vi "forward difference (i32).vi"(3 "Y":i32[](array[numeric])) -> (1 "Y(i+1)-Y(i)":i32[](array[numeric]))   [LabVIEW 2009, in "common.lvlib"]
uses:
  common.lvlib
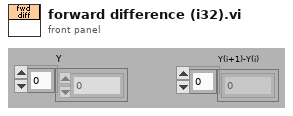
[diagram p1: front panel]
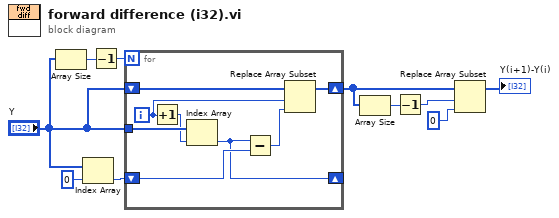
[diagram p0: block diagram]
diagram:
  n1 = Array Size(array="Y") -> (size(s)=w10:i32)
  n2 = Index Array(array="Y", index=0) -> (element=w7:i32)
  n3 = Decrement(x=w10) -> (x-1=w9:i32)
  n4 = for {
    N: w9 -> [_]
    tunnel: "Y" -> [w18]
    shift-right: [w15] -> _
    shift-left: w7 -> [w16]
    shift-right: [w11] -> w4
    shift-left: "Y" -> [w12]
    i -> [w13]
    n5 = Increment(x=w13) -> (x+1=w17:i32)
    n6 = Index Array(array=w18, index=w17) -> (element=w15:i32)
    n7 = Subtract(x=w15, y=w16) -> (x-y=w14:i32)
    n8 = Replace Array Subset(array=w12, new element=w14, index=w13) -> (w11:i32[])
  }
  n9 = Array Size(array=w4) -> (size(s)=w3:i32)
  n10 = Decrement(x=w3) -> (x-1=w2:i32)
  n11 = Replace Array Subset(array=w4, new element=0 ("new element/subarray"), index=w2) -> (→"Y(i+1)-Y(i)":i32[])
